vi "Get Queue Error.vi"(8 "error in (no error)":errorcluster) -> (0 "error out":errorcluster, 2 "Queues":T1, 3 "Error Queue":refnum<queue>)   [LabVIEW 2023, in "Error Handling.lvlib"]
uses:
  Error Handling.lvlib
  Internal Communication/Controls/Queues Control.ctl
  Downloads/ATM (100528-01)/ATM (100528-01)/Omi-One Solution/Inner Process Communication/States Queues FGV.ctl
  Downloads/ATM (100528-01)/ATM (100528-01)/Omi-One Solution/Inner Process Communication/Innes Process Communication.lvlib
  Internal Communication/Internal Communication.lvlib
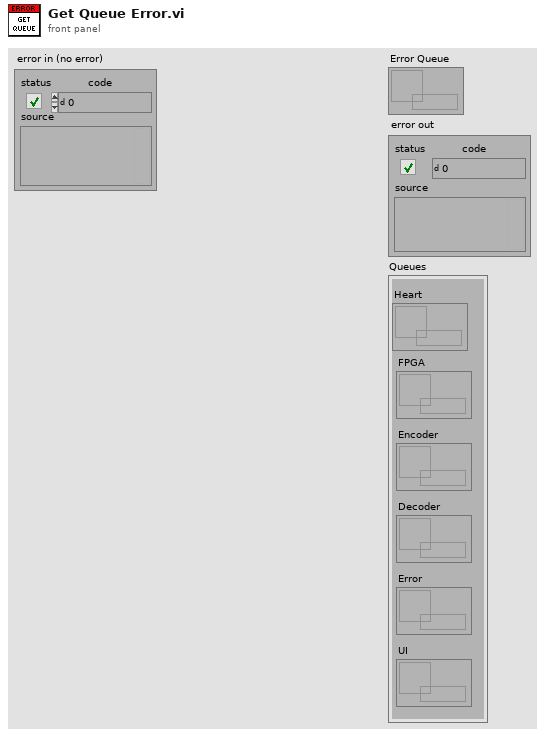
[diagram p1: front panel]
types:
  T1 = typedef "Internal Communication.lvlib/Queues Control.ctl" = cluster{"Heart":refnum<queue>, "FPGA":refnum<queue>, "Encoder":refnum<queue>, "Decoder":refnum<queue>, "Error":refnum<queue>, "UI":refnum<queue>}
  T2 = typedef "Innes Process Communication.lvlib/States Queues FGV.ctl" = enum16{"Create Queues", "Get Queues", "Destroy Queues"}
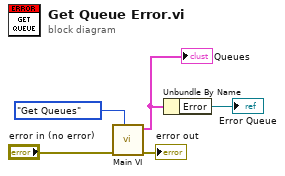
[diagram p0: block diagram]
diagram:
  n1 = call "Main VI.vi"("Enum"=States_Queues_FGV."Get Queues", "error in (no error)"="error in (no error)") -> ("error out"=→"error out":errorcluster, "Queues"=w1:T1)  [unwired: 8 in]
  "Queues" <- w1
  n2 = Unbundle By Name(w1) -> ("Error"=→"Error Queue":refnum<queue>)
